vi "NI_Gmath.Eval Single-Variable Array CUSTOM.vi"(6 "New Formulas":bool, 8 "error in (no error)":errorcluster, 9 "Prev Parsed Formula":cluster{"Table":i32[][], "Y Values":dbl[]} {"Y Values" format="%.2f"}, 10 "formula in":string, 11 "X Values":dbl[](array[numeric]) format="%0.2f") -> (0 "error out":errorcluster, 1 "Parsed Formula":cluster{"Table":i32[][], "Y Values":dbl[]}, 3 "Y Values":dbl[](array[numeric]) format="%0.2f")   [LabVIEW 2014, in "RT - Analysis.lvlib"]
doc: "This custom version allows for a previous parsed string's cluster to be used instead of the string input.\n\nCalculates an array of function values at given points in a given interval by y[i] = f(x[i]) for i = 1, ...n, where f is the 1D function given by the user formula."
uses:
  RT - Analysis.lvlib
  <vilib>/gmath/parser.llb/Three Register Calculation.VI
  <vilib>/gmath/NI_Gmath.lvlib
panel:
  # "Example:\n\n formula: x*sin(x)\n X Values: (1.0,1.56,3.14)"
  # "operator"
  # "register1"
  # "register2"
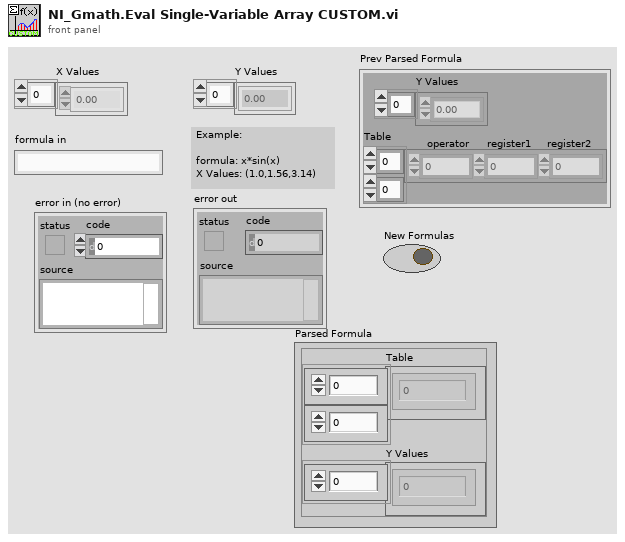
[diagram p1: front panel]
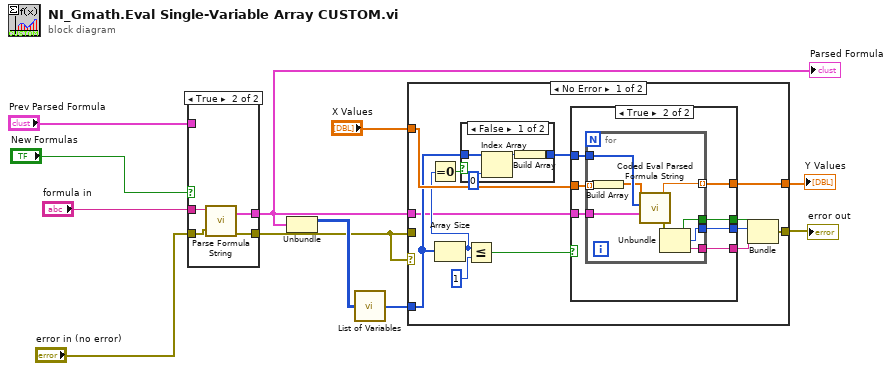
[diagram p0: block diagram]
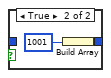
[diagram p3: hidden frame]
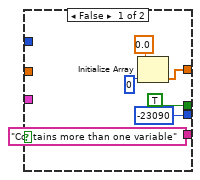
[diagram p4: hidden frame]
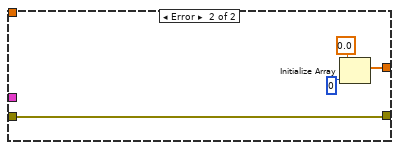
[diagram p5: hidden frame]
diagram:
  n1 = case shown="True" "New Formulas" {
    tunnel: "formula in" -> [_ w17]
    tunnel: "error in (no error)" -> [w12 w16]
    tunnel: [w12 w15] -> w4
    tunnel: [w13 w14] -> w3
    tunnel: "Prev Parsed Formula" -> [w13 _]
    frame False {
    }
    frame True {
      n2 = call <vilib>:"Parse Formula String.vi"("error in (no error)"=w16, "formula"=w17) -> ("error out"=w15:errorcluster, "Parsed Formula"=w14:cluster{"Table":i32[][], "Y Values":dbl[]})
    }
  }
  "Parsed Formula" <- w3
  n3 = Unbundle(w3) -> ("Table"=w5:i32[][])  [unwired: 1 out]
  n4 = call <vilib>:"List of Variables.vi"("Table"=w5) -> ("List of variables"=w7:i32[])
  n5 = case shown="No Error" w4 {
    tunnel: [w30 w59] -> w8
    tunnel: w4 -> [_ w62]
    tunnel: w7 -> [w26 _]
    tunnel: "X Values" -> [w27 _]
    tunnel: [w19 w62] -> w11
    tunnel: w3 -> [w18 _]
    frame No Error {
      n6 = Array Size(array=w26) -> (size(s)=w24:i32)
      n7 = Equal To 0?(x=w24) -> (x = 0?=w23:bool)
      n8 = case shown="False" w23 {
        tunnel: [w32 w36] -> w25
        tunnel: w26 -> [w31 _]
        frame False {
          n9 = Index Array(array=w31, index=0) -> (element=w33:i32)
          n10 = Build Array(w33) -> (w32:i32[])
        }
        frame True {
          n11 = Build Array(1001) -> (w36:i32[])
        }
      }
      n12 = Less Or Equal?(x=w24, y=1) -> (x <= y?=w28:bool)
      n13 = case shown="True" w28 {
        tunnel: w27 -> [_ w49]
        tunnel: [w37 w48] -> w30
        tunnel: w25 -> [_ w47]
        tunnel: [TRUE w46] -> w22
        tunnel: [-23090 w45] -> w21
        tunnel: ["Contains more than one variable" w44] -> w20
        tunnel: w18 -> [_ w43]
        frame False {
          n14 = Initialize Array(0.0, 0) -> (w37:dbl[])
        }
        frame True {
          n15 = for {
            tunnel: w47 -> [w52]
            tunnel: [w58] -> w48 mode=indexing
            tunnel: w49 -> [w57] mode=indexing
            tunnel: [w55] -> w46
            tunnel: [w54] -> w45
            tunnel: [w53] -> w44
            tunnel: w43 -> [w50]
            n16 = Build Array(w57) -> (w51:dbl[])
            n17 = call <vilib>:"Coded Eval Parsed Formula String.vi"("Parsed Formula"=w50, "Variables"=w52, "X Values"=w51) -> ("error out"=w56:errorcluster, "y value"=w58:dbl)  [unwired: 1 in]
            n18 = Unbundle(w56) -> ("status"=w55:bool, "code"=w54:i32, "source"=w53:string)
          }
        }
      }
      n19 = Bundle("status"=w22, "code"=w21, "source"=w20) -> (w19:errorcluster)  [unwired: 1 in]
    }
    frame Error {
      n20 = Initialize Array(0.0, 0) -> (w59:dbl[])
    }
  }
  "Y Values" <- w8
  "error out" <- w11
